vi "Configure.vi"(8 "error in (no error)":errorcluster, 11 "Stage_MadCityLabMicro in":refnum<class "Stage_MadCityLabMicro.lvclass">) -> (0 "error out":errorcluster, 3 "Stage_MadCityLabMicro out":refnum<class "Stage_MadCityLabMicro.lvclass">)   [LabVIEW 2020, in "Stage_MadCityLabMicro.lvlib" / "Stage_MadCityLabMicro.lvclass"]
uses:
  Stage_MadCityLabMicro.lvclass
  E:/Development/DevHardSoftware/MMicroscopyAF/Model/HAL Layer/Component/Device/Device/Device.lvclass
  HAL Layer/Component/Stage/Stage/Stage.lvclass
  HAL Layer/Component/Device/Device/Device.lvclass
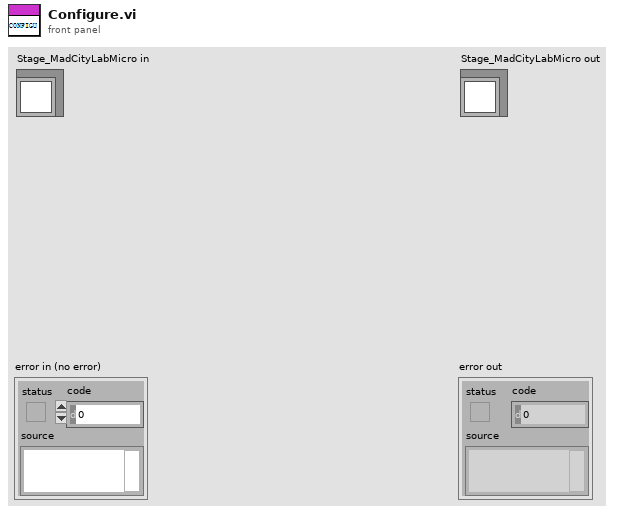
[diagram p1: front panel]
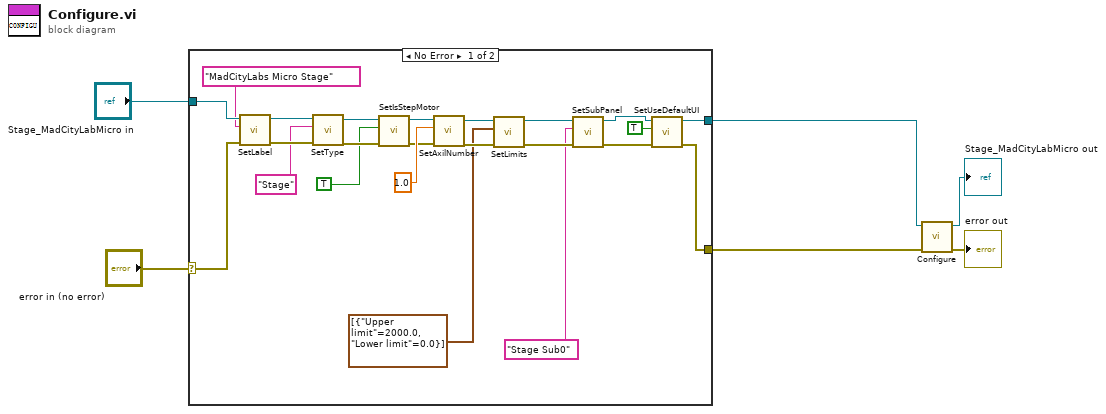
[diagram p0: block diagram]
diagram:
  n1 = case shown="No Error" "error in (no error)" {
    selector: "error in (no error)" -> [w28 w31]
    tunnel: [w13 w31] -> w1
    tunnel: [w12 w30] -> w2
    tunnel: "Stage_MadCityLabMicro in" -> [w29 w30]
    frame No Error {
      n2 = call-dynamic "SetLabel.vi"("error in (no error)"=w28, "Label"="MadCityLabs Micro Stage", "Device in"=w29) -> ("error out"=w25:errorcluster, "Device out"=w26:refnum<class "Stage_MadCityLabMicro.lvclass">)  [unwired: 7 in]
      n3 = call-dynamic "SetType.vi"("error in (no error)"=w25, "Type"="Stage", "Device in"=w26) -> ("error out"=w16:errorcluster, "Device out"=w18:refnum<class "Stage_MadCityLabMicro.lvclass">)  [unwired: 7 in]
      n4 = call-dynamic "SetIsStepMotor.vi"("error in (no error)"=w16, "StepMotor?"=TRUE, "Stage in"=w18) -> ("error out"=w17:errorcluster, "Stage out"=w19:refnum<class "Stage_MadCityLabMicro.lvclass">)  [unwired: 7 in]
      n5 = call-dynamic "SetAxilNumber.vi"("error in (no error)"=w17, "Axil Number"=1.0, "Stage in"=w19) -> ("error out"=w21:errorcluster, "Stage out"=w22:refnum<class "Stage_MadCityLabMicro.lvclass">)  [unwired: 7 in]
      n6 = call-dynamic "SetLimits.vi"("error in (no error)"=w21, "Limits"=cluster{"Upper limit":dbl, "Lower limit":dbl}[] [{"Upper limit"=2000.0, "Lower limit"=0.0}], "Stage in"=w22) -> ("error out"=w20:errorcluster, "Stage out"=w9:refnum<class "Stage_MadCityLabMicro.lvclass">)  [unwired: 7 in]
      n7 = call-dynamic "SetSubPanel.vi"("error in (no error)"=w20, "Sub Panel"="Stage Sub0", "Device in"=w9) -> ("error out"=w10:errorcluster, "Device out"=w8:refnum<class "Stage_MadCityLabMicro.lvclass">)  [unwired: 7 in]
      n8 = call "SetUseDefaultUI.vi"("error in (no error)"=w10, "Use Default UI?"=TRUE, "Device in"=w8) -> ("error out"=w13:errorcluster, "Device out"=w12:refnum<class "Stage_MadCityLabMicro.lvclass">)  [unwired: 7 in]
    }
    frame Error {
    }
  }
  n9 = call-parent "Configure.vi"("error in (no error)"=w1, "Device in"=w2) -> ("error out"=→"error out":errorcluster, "Device out"=→"Stage_MadCityLabMicro out":refnum<class "Stage_MadCityLabMicro.lvclass">)  [unwired: 8 in]
